vi "Teardown.vi"(11 "Actor in":refnum<class "Actor.lvclass">) -> (2 "Teardown?":bool, 3 "Actor out":refnum<class "Actor.lvclass">)   [LabVIEW 2021, in "jettl.lvlib" / "Actor.lvclass"]
uses:
  Actor.lvclass
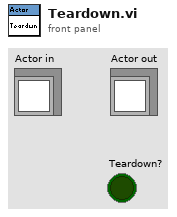
[diagram p1: front panel]
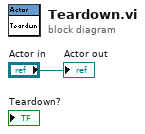
[diagram p0: block diagram]
diagram:
  "Actor out" <- "Actor in"
